vi "Auto - Total Distance (SubVI).vi"(6 "Auto Y":dbl, 7 "Auton State In":i32, 8 "disabledRunning":bool, 9 "Auto X":dbl, 10 "Pose Translation Y":dbl, 11 "Pose Translation X":dbl) -> (0 "distanceLeftToDrivenInThisStep":dbl, 3 "totalDistanceToDriveInThisStep":dbl)   [LabVIEW 2020]
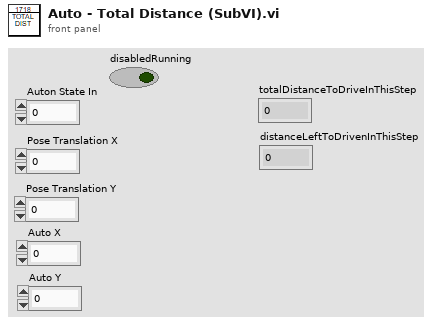
[diagram p1: front panel]
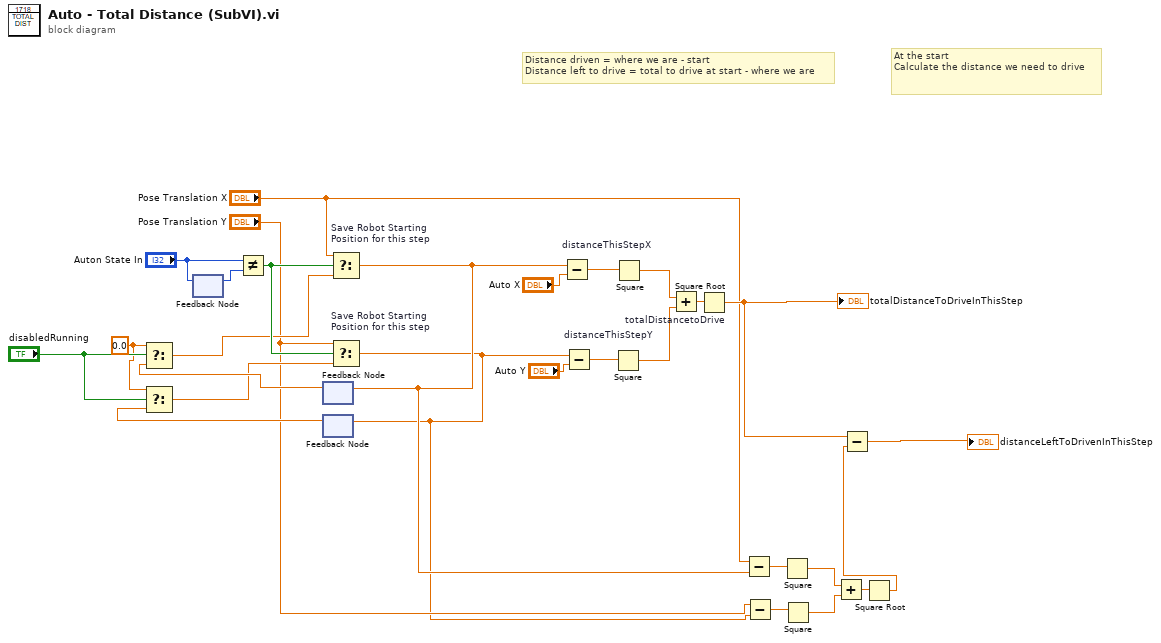
[diagram p0: block diagram]
diagram:
  w15 = 0.0 ("t")
  # "At the start\nCalculate the distance we need to drive"
  # "Distance driven = where we are - start\nDistance left to drive = total to drive at start - where we are"
  n1 = feedback #1() -> (w23:i32)  [unwired: 1 in]
  n2 = feedback-in #1("Auton State In") -> ()
  n3 = Not Equal?(x="Auton State In", y=w23) -> (x != y?=w24:bool)
  n4 = feedback #2() -> (w14:dbl)  [unwired: 1 in]
  n5 = Select(t=w15, s="disabledRunning", f=w14) -> (s? t:f=w13:dbl)
  n6 = feedback #3() -> (w16:dbl)  [unwired: 1 in]
  n7 = Select(t=w15, s="disabledRunning", f=w16) -> (s? t:f=w12:dbl)
  n8 = Select "Save Robot Starting\nPosition for this step"(t="Pose Translation X", s=w24, f=w13) -> (s? t:f=w3:dbl)
  n9 = feedback-in #2(w3) -> ()
  n10 = Select "Save Robot Starting \nPosition for this step"(t="Pose Translation Y", s=w24, f=w12) -> (s? t:f=w2:dbl)
  n11 = feedback-in #3(w2) -> ()
  n12 = Subtract "distanceThisStepX"(x=w3, y="Auto X") -> (x-y=w11:dbl)
  n13 = Subtract "distanceThisStepY"(x=w2, y="Auto Y") -> (x-y=w10:dbl)
  n14 = Square(x=w10) -> (x^2=w27:dbl)
  n15 = Square(x=w11) -> (x^2=w26:dbl)
  n16 = Add(x=w26, y=w27) -> (x+y=w28:dbl)
  n17 = Square Root "totalDistancetoDrive"(x=w28) -> (sqrt(x)=w9:dbl)
  "totalDistanceToDriveInThisStep" <- w9
  n18 = Subtract(x="Pose Translation X", y=w3) -> (x-y=w7:dbl)
  n19 = Subtract(x="Pose Translation Y", y=w2) -> (x-y=w6:dbl)
  n20 = Square(x=w7) -> (x^2=w20:dbl)
  n21 = Square(x=w6) -> (x^2=w19:dbl)
  n22 = Add(x=w20, y=w19) -> (x+y=w18:dbl)
  n23 = Square Root(x=w18) -> (sqrt(x)=w8:dbl)
  n24 = Subtract(x=w9, y=w8) -> (x-y=→"distanceLeftToDrivenInThisStep":dbl)
